vi "myRIO Main v2.vi"() -> ()   [LabVIEW 2014]
uses:
  Type Defs/VL6180 states.ctl
  <vilib>/Platform/TimedLoop/XDataNode/timing_clust.ctl
  <vilib>/Platform/TimedLoop/XDataNode/nitl_modes.ctl
  <vilib>/Platform/TimedLoop/XDataNode/wakeup.ctl
  Type Defs/VL6180 Resource.ctl
  <vilib>/myRIO/Instrument Drivers/Onboard IO/DIO/typedefs/DIO Reference.ctl
  <vilib>/myRIO/Common/Instrument Driver Framework/Utilities/typedefs/myRIO Generic Hardware Reference.ctl
  <vilib>/myRIO/Common/Instrument Driver Framework/Utilities/typedefs/Hardware Version Enum.ctl
  <vilib>/myRIO/Common/Instrument Driver Framework/Utilities/typedefs/myRIO v1.0 Reference.ctl
  <vilib>/myRIO/Common/Instrument Driver Framework/Utilities/typedefs/Generic FPGA Reference.ctl
  <vilib>/myRIO/Common/Instrument Driver Framework/myRIO v1.0/DIO/typedefs/DIO Channels List.ctl
  <vilib>/myRIO/Common/Instrument Driver Framework/myRIO v1.0/DIO/typedefs/DIO Channels Enum.ctl
  <vilib>/userdefined/High Color/nirio_resource_hc.ctl
  <vilib>/myRIO/Instrument Drivers/Onboard IO/AI/typedefs/AI Reference.ctl
  <vilib>/myRIO/Common/Instrument Driver Framework/myRIO v1.0/AI/typedefs/AI Channels List.ctl
  <vilib>/myRIO/Common/Instrument Driver Framework/myRIO v1.0/AI/typedefs/AI Channels Enum.ctl
  <vilib>/myRIO/Common/Instrument Driver Framework/Utilities/typedefs/Analog Scaling Constants List.ctl
  <vilib>/myRIO/Common/Instrument Driver Framework/Utilities/typedefs/Analog Scaling Constants.ctl
  <vilib>/myRIO/Common/Instrument Driver Framework/Utilities/vis/Is FPGA Ref Available.vi
  <vilib>/myRIO/Common/Instrument Driver Framework/myRIO v1.0/DIO/vis/myRIO v1.1 Open DIO.vi
  <vilib>/myRIO/Instrument Drivers/Onboard IO/DIO/vis/Read.vi
  <vilib>/myRIO/Common/Instrument Driver Framework/myRIO v1.0/AI/vis/myRIO v1.1 Open AI.vi
  <vilib>/myRIO/Instrument Drivers/Onboard IO/AI/vis/Read.vi
  <vilib>/myRIO/Instrument Drivers/Onboard IO/DIO/vis/Write.vi
  <vilib>/MakerHub/LINX/Public/Peripherals/Digital/Digital Write 1 Chan.vi
  <vilib>/myRIO/Common/Instrument Driver Framework/Utilities/vis/Validate Channels.vi
  <vilib>/myRIO/Common/Instrument Driver Framework/myRIO v1.0/DIO/vis/myRIO v1.0 Reserve DIO.vi
  <vilib>/myRIO/Common/Instrument Driver Framework/myRIO v1.0/AI/vis/myRIO v1.0 Reserve AI.vi
  <vilib>/MakerHub/LINX/Public/Peripherals/Digital/Digital Write N Chans.vi
  <vilib>/myRIO/Common/Instrument Driver Framework/myRIO v1.0/Resource Manager/vis/myRIO v1.0 Reserve Channel List.vi
  <vilib>/myRIO/Common/Instrument Driver Framework/myRIO v1.0/DIO/vis/myRIO v1.0 Build MUX Configuration DIO.vi
  <vilib>/myRIO/Common/Instrument Driver Framework/myRIO v1.0/AI/vis/myRIO v1.0 Build MUX Configuration AI.vi
  <vilib>/MakerHub/LINX/Private/Local IO/LinxDigitalWrite.vi
  <vilib>/MakerHub/LINX/Public/Utilities/Check Channel.vi
  <vilib>/myRIO/Common/Instrument Driver Framework/myRIO v1.0/Resource Manager/vis/myRIO v1.0 Reserve Channel.vi
  <vilib>/myRIO/Common/Instrument Driver Framework/myRIO v1.0/Resource Manager/vis/myRIO v1.0 Unreserve Channel.vi
  <vilib>/myRIO/Common/Instrument Driver Framework/myRIO v1.0/Resource Manager/vis/myRIO v1.0 Create Configuration List.vi
  <vilib>/MakerHub/LINX/Private/myRIO/Utilities/Get DIO Channel Name.vi
  <vilib>/myRIO/Common/Instrument Driver Framework/myRIO v1.0/Resource Manager/vis/myRIO v1.0 Build Mutex Name.vi
  <vilib>/Utility/VariantDataType/GetNumericInfo.vi
  <vilib>/Utility/error.llb/Error Cluster From Error Code.vi
  <vilib>/myRIO/Common/Instrument Driver Framework/myRIO v1.0/myRIO v1.1 Open.vi
  <vilib>/myRIO/Common/Instrument Driver Framework/myRIO v1.0/AI/vis/myRIO v1.0 Get Scaling Constants AI.vi
  <vilib>/myRIO/Common/Instrument Driver Framework/Utilities/vis/IO Manager.vi
  <vilib>/myRIO/Common/Instrument Driver Framework/Utilities/vis/Configuration Manager.vi
  <vilib>/myRIO/Common/Instrument Driver Framework/myRIO v1.0/myRIO v1.0 Close.vi
  <vilib>/myRIO/Common/Instrument Driver Framework/myRIO v1.0/AI/vis/myRIO v1.0 Read AI.vi
  <vilib>/myRIO/Common/Instrument Driver Framework/myRIO v1.0/Resource Manager/vis/myRIO v1.0 Configure IO.vi
  <vilib>/myRIO/Common/Instrument Driver Framework/myRIO v1.0/DIO/vis/myRIO v1.0 Write DIO.vi
  <vilib>/MakerHub/LINX/Public/Utilities/Open Local.vi
  <vilib>/MakerHub/LINX/Private/Utilties/Generate Error.vi
  <vilib>/myRIO/Instrument Drivers/Onboard IO/DIO/vis/Smart Open.vi
  <vilib>/myRIO/Common/Instrument Driver Framework/myRIO v1.0/DIO/vis/myRIO v1.0 Read DIO.vi
  <vilib>/myRIO/Express VI/Onboard IO/AI/AI Express VI.xnode
  <vilib>/myRIO/Instrument Drivers/Onboard IO/AI/vis/myRIO AI Open.xnode
  <vilib>/myRIO/Express VI/Onboard IO/DO/DO Express VI.xnode
  <vilib>/myRIO/Instrument Drivers/Onboard IO/DIO/vis/myRIO DIO Open.xnode
  <vilib>/platform/TimedLoop/XDataNode/XDataNode.xnode
  <vilib>/myRIO/Express VI/Onboard IO/DI/DI Express VI.xnode
  <vilib>/MakerHub/LINX/LMH-LINX.lvlib
  <vilib>/Platform/TimedLoop/XDataNode/XDNodeRunTimeDep.lvlib
  <vilib>/myRIO/Instrument Drivers/Onboard IO/DIO/DIO.lvlib
  <vilib>/myRIO/Express VI/Onboard IO/I2C/I2C Express VI.xnode
  <vilib>/myRIO/Instrument Drivers/Onboard IO/I2C/vis/Configure.vi
  <vilib>/myRIO/Instrument Drivers/Onboard IO/I2C/I2C.lvlib
  <vilib>/myRIO/Instrument Drivers/Onboard IO/I2C/vis/Write.vi
  <vilib>/myRIO/Instrument Drivers/Onboard IO/I2C/typedefs/I2C Transfer Rate.ctl
  <vilib>/myRIO/Instrument Drivers/Onboard IO/I2C/typedefs/I2C User Configuration.ctl
  <vilib>/myRIO/Instrument Drivers/Onboard IO/I2C/typedefs/I2C Configuration.ctl
  <vilib>/myRIO/Common/Instrument Driver Framework/myRIO v1.0/I2C/typedefs/I2C Channels Enum.ctl
  <vilib>/myRIO/Instrument Drivers/Onboard IO/I2C/typedefs/I2C Reference.ctl
  <vilib>/myRIO/Instrument Drivers/Onboard IO/I2C/vis/myRIO I2C Open.xnode
  <vilib>/myRIO/Common/Instrument Driver Framework/myRIO v1.0/I2C/vis/myRIO v1.1 Open I2C.vi
  <vilib>/myRIO/Instrument Drivers/Onboard IO/I2C/vis/Read.vi
  <vilib>/myRIO/Instrument Drivers/Onboard IO/AI/AI.lvlib
panel:
  out "5V Regulator":dbl(knob) scale=0.0..6.0
  in  "Sensor Power":bool
  out "Laser Error":bool
  in  "Reset":bool
  in  "Stop":bool
  in  "Wait (ms)":u32=10
  out "ToF Loop Rate":u32
  in  "Speed Read":bool
  out "Attempts":i32
  out "Sensor Error Code":u8
  in  "Attempts before Timeout":u16=10
  in  "delay":u32=500
  in  "I2C Channel":u8
  out "Sensors Online":bool[](array[boolean])
  in  "# of sensors":i32=5
  out "Status":string
  in  "Track Location":dbl(slide) scale=0.0..5000.0
  out "Structure\nStress":dbl(slide) scale=2.4..2.6
  out "Track Position":T1
  out "Battery (Primary)":dbl(slide) scale=0.0..100.0 scale format="%.1f%"
  out "Current":dbl(knob) scale=0.0..1.0
  out "IMU":T2 {"Magnetometer"."Z" scale=0.0..100.0; "Magnetometer"."Y" scale=0.0..100.0; "Magnetometer"."X" scale=0.0..100.0; "Gyroscope"."R" scale=0.0..100.0; "Gyroscope"."Y" scale=0.0..100.0; "Gyroscope"."P" scale=0.0..100.0; "Accelerometer"."Z" scale=0.0..100.0; "Accelerometer"."Y" scale=0.0..100.0; "Accelerometer"."X" scale=0.0..100.0}
  out "Voltage":dbl(knob) scale=0.0..12.0
  out "Gap 4":u8(slide) scale=0.0..100.0
  out "Gap 3":u8(slide) scale=0.0..100.0
  out "Rail Gap 2":u8(slide) scale=0.0..100.0
  out "Gap 2":u8(slide) scale=0.0..100.0
  out "Temp 2":dbl(slide) scale=0.0..100.0
  out "Temp 1":dbl(slide) scale=0.0..100.0
  out "Rail Gap 1":u8(slide) scale=0.0..100.0
  out "Gap 1":u8(slide) scale=0.0..100.0
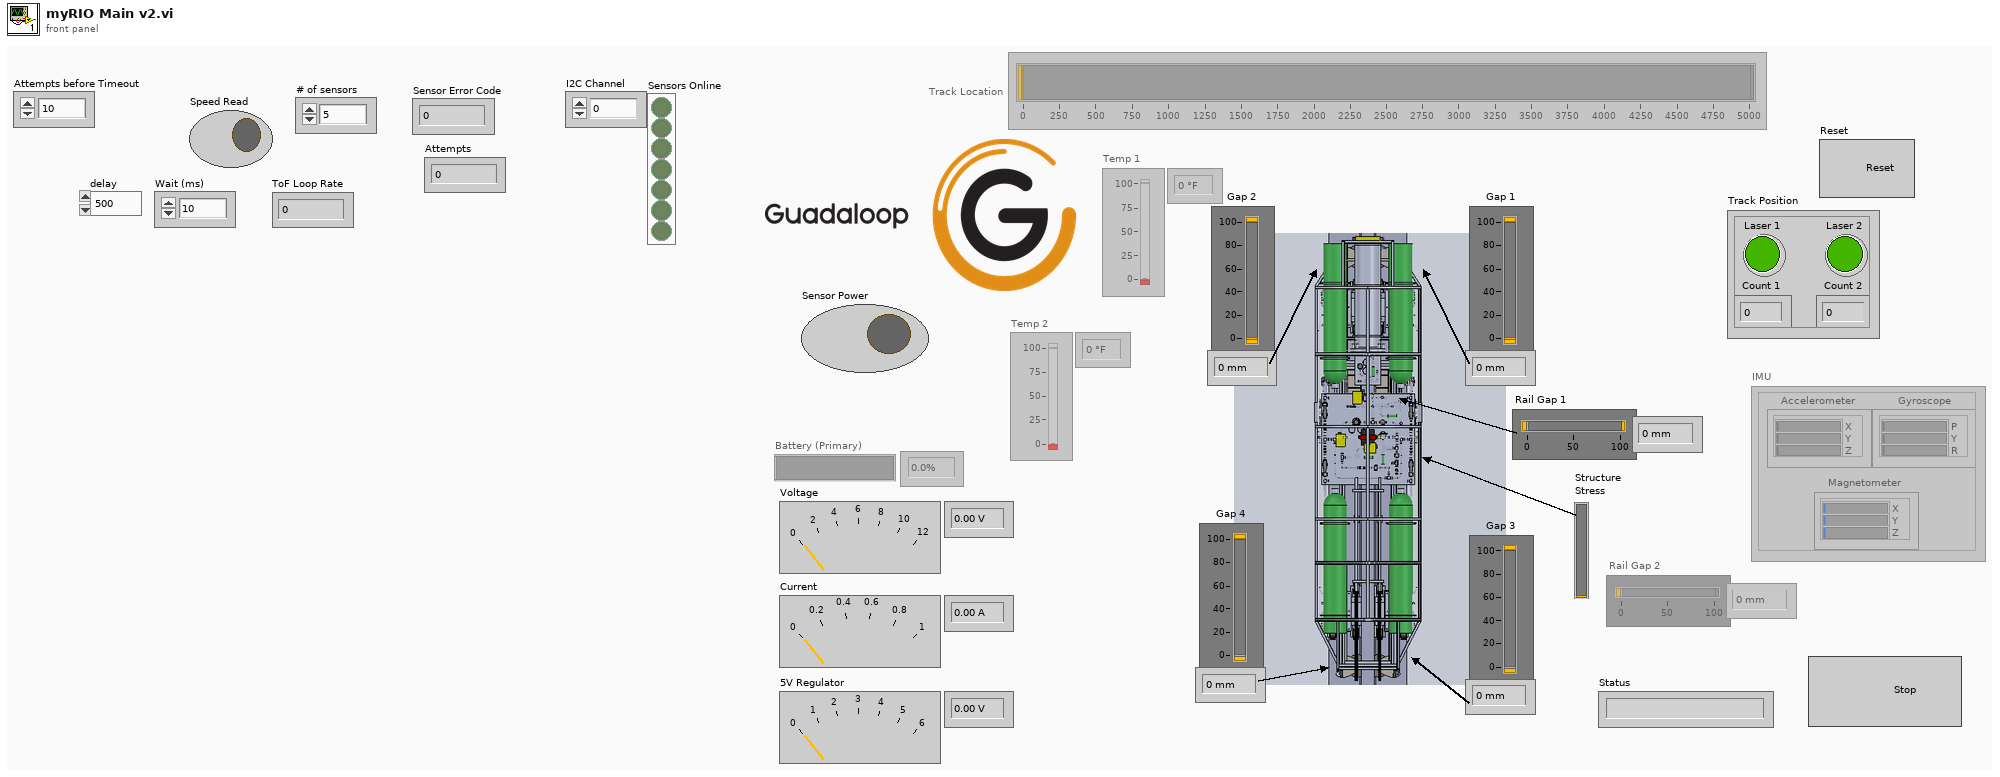
[diagram p1: front panel]
types:
  T1 = cluster{"Laser 1":bool, "Count 1":u32, "Laser 2":bool, "Count 2":u32}
  T2 = cluster{"Accelerometer":cluster{"X":u8, "Y":u8, "Z":u8}, "Gyroscope":cluster{"P":u8, "Y":u8, "R":u8}, "Magnetometer":cluster{"X":u8, "Y":u8, "Z":u8}}
  T3 = typedef "VL6180 states.ctl" = enum16{"Ping All", "Initialize", "Read"}
  T4 = typedef "XDNodeRunTimeDep.lvlib/timing_clust.ctl" = cluster{"Expected End [f-1]":u64, "Actual End [f-1]":u64, "Finished Late? [f-1]":bool, "Expected End [i-1]":u64, "Actual End [i-1]":u64, "Finished Late? [i-1]":bool, "Expected Start [i]":u64, "Actual Start [i]":u64, "Expected Start [f]":u64, "Actual Start [f]":u64, "Source Name":string, "Structure Name":string, "Period":i64, "Deadline":i64, "Offset":i64, "Start":i64, "Priority":i32, "Timeout":i32, "Mode":T5, "Wakeup Reason":T6, "Error":errorcluster, "Source Type":string, "Secondary Source Type":string, "Global End Time":u64, "Global Start Time":u64, "Frame Duration":u64, "Iteration Duration":u64, "Assigned CPU":i32, "I/O Scan Engine Mode":u32}
  T5 = typedef "XDNodeRunTimeDep.lvlib/nitl_modes.ctl" = enum32{"No Change", "Process missed periods, maintain original phase", "Discard missed periods, maintain original phase", "Process missed periods, ignore original phase", "Discard missed periods, ignore original phase"}
  T6 = typedef "XDNodeRunTimeDep.lvlib/wakeup.ctl" = enum32{"Normal", "Aborted", "Asynchronous wakeup", "Timing source error", "Timed loop error", "Timeout"}
  T7 = typedef "LMH-LINX.lvlib/LINX Ref.ctl" = cluster{"IO":T8, "Interface":T9, "LINX Device Config":T10}
  T8 = typedef "LMH-LINX.lvlib/Platform.ctl" = enum16{"Remote", "Local"}
  T9 = typedef "LMH-LINX.lvlib/Interface.ctl" = enum16{"Serial", "TCP"}
  T10 = typedef "LMH-LINX.lvlib/Device.lvlib/LINX Device Config.ctl" = cluster{"Interface":T9, "COM Port":refnum<visa-resource-name>, "TCP Configuration":T11, "Device Family":u8, "Device ID":u8, "Device Name":string, "TCP Ref":refnum<k5>, "Channels":T12}
  T11 = typedef "LMH-LINX.lvlib/Device.lvlib/TCP Config.ctl" = cluster{"IP Address":string, "Port":u16}
  T12 = typedef "LMH-LINX.lvlib/Channels.ctl" = cluster{"DI":u8[], "DO":u8[], "AI":u8[], "AO":u8[], "PWM":u8[], "QE":u8[], "UART":u8[], "I2C 2":u8[], "SPI":u8[], "CAN":u8[], "Servo":u8[], "AI Ref (V)":dbl, "AI Resolution (Bits)":u8, "AO Ref (V)":dbl, "AO Resolution (Bits)":u8}
  T13 = typedef "DIO.lvlib/DIO Reference.ctl" = cluster{"myRIO Reference":T14, "DIO Channels List":T18}
  T14 = typedef "myRIO Generic Hardware Reference.ctl" = cluster{"myRIO Model":T15, "myRIO Hardware Reference":T16}
  T15 = typedef "Hardware Version Enum.ctl" = enum16{"Unknown", "myRIO-1900", "myRIO-1950"}
  T16 = typedef "myRIO v1.0 Reference.ctl" = cluster{"Generic FPGA Reference":T17, "Allow multiple opens":bool}
  T17 = typedef "Generic FPGA Reference.ctl" = refnum<k20>
  T18 = typedef "DIO Channels List.ctl" = T19[]
  T19 = typedef "DIO Channels Enum.ctl" = enum16{"Not Connected", "C/DIO0", "C/DIO1", "C/DIO2", "C/DIO3", "C/DIO4", "C/DIO5", "C/DIO6", "C/DIO7", "A/DIO0", "A/DIO1", "A/DIO2", "A/DIO3", "A/DIO4", "A/DIO5", "A/DIO6", "A/DIO7", "A/DIO8", "A/DIO9", "A/DIO10", "A/DIO11", "A/DIO12", "A/DIO13", "A/DIO14", "A/DIO15", "B/DIO0", "B/DIO1", "B/DIO2", "B/DIO3", "B/DIO4", "B/DIO5", "B/DIO6", "B/DIO7", "B/DIO8", "B/DIO9", "B/DIO10", "B/DIO11", "B/DIO12", "B/DIO13", "B/DIO14", "B/DIO15", "LED0", "LED1", "LED2", "LED3", "Button0"}
  T20 = typedef "nirio_resource_hc.ctl" = tag
  T21 = typedef "VL6180 Resource.ctl" = cluster{"I2C Channel":u8, "I2C Slave Address":u8, "Online":bool}
  T22 = typedef "I2C.lvlib/I2C Reference.ctl" = cluster{"myRIO Reference":T14, "I2C Channels Enum":T23, "I2C Configuration":T24}
  T23 = typedef "I2C Channels Enum.ctl" = enum16{"Not Connected", "A/I2C", "B/I2C"}
  T24 = typedef "I2C.lvlib/I2C Configuration.ctl" = cluster{"I2C Transfer Rate":T25}
  T25 = typedef "I2C.lvlib/I2C Transfer Rate.ctl" = enum16{"Standard mode (100 kbps)", "Fast mode (400 kbps)"}
  T26 = typedef "I2C.lvlib/I2C User Configuration.ctl" = cluster{"I2C Transfer Rate":T25}
  T27 = typedef "AI.lvlib/AI Reference.ctl" = cluster{"myRIO Reference":T14, "AI Channels List":T28, "AI Scaling Constants List":T30}
  T28 = typedef "AI Channels List.ctl" = T29[]
  T29 = typedef "AI Channels Enum.ctl" = enum16{"Not Connected", "AudioIn/Left", "AudioIn/Right", "C/AI0", "C/AI1", "A/AI0", "A/AI1", "A/AI2", "A/AI3", "B/AI0", "B/AI1", "B/AI2", "B/AI3"}
  T30 = typedef "Analog Scaling Constants List.ctl" = T31[]
  T31 = typedef "Analog Scaling Constants.ctl" = cluster{"LSB Weight (Volts)":dbl, "Offset (Volts)":dbl, "Signed?":bool}
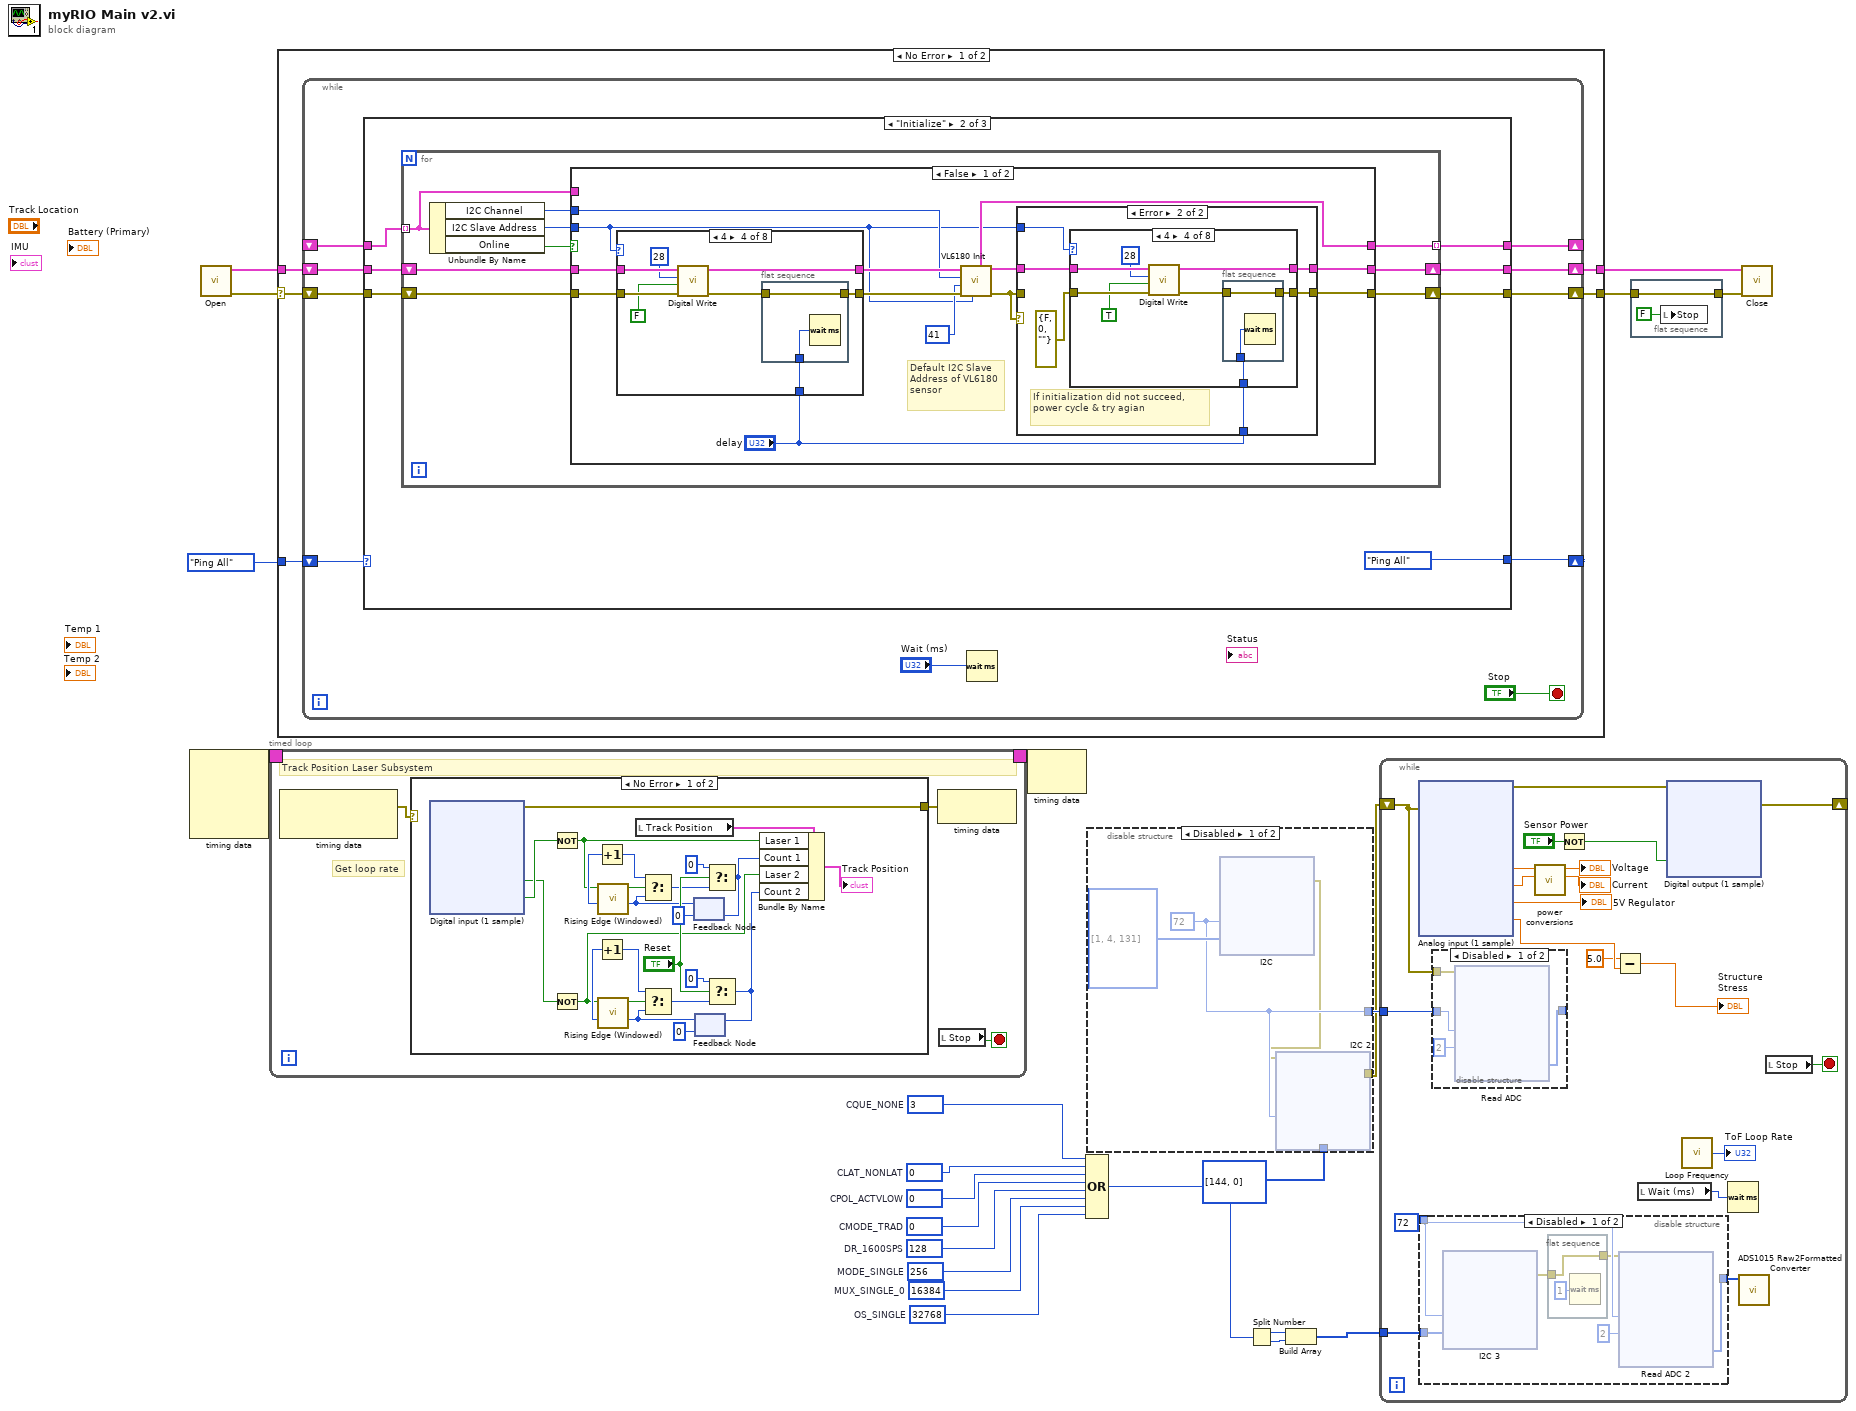
[diagram p0: block diagram]
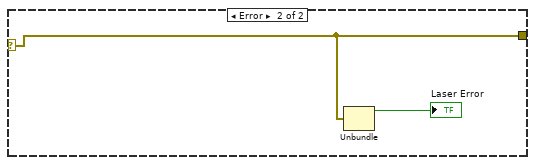
[diagram p5: hidden frame]
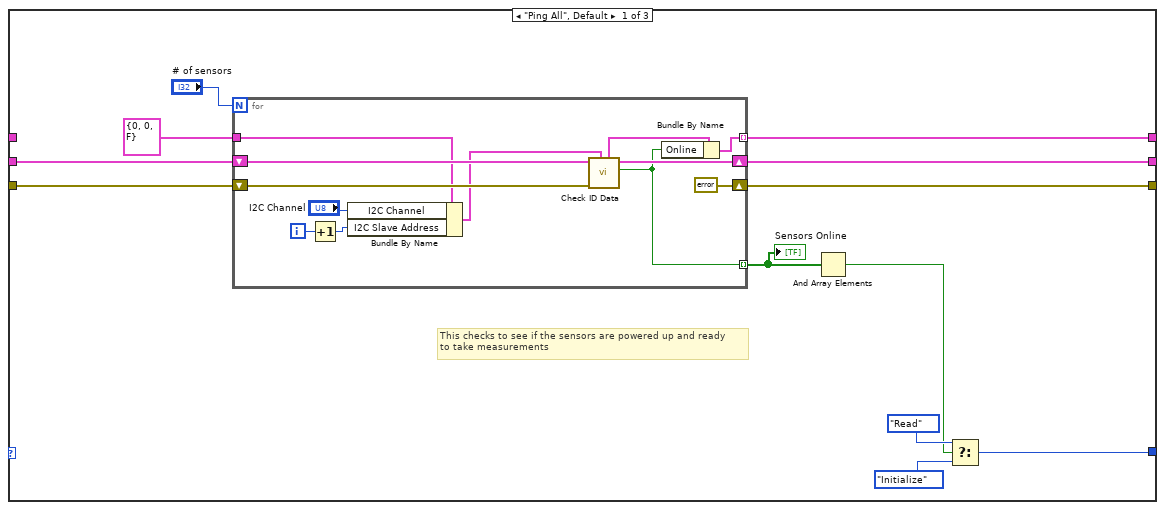
[diagram p6: hidden frame]
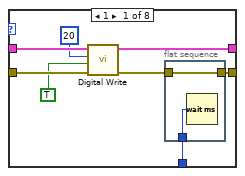
[diagram p8: hidden frame]
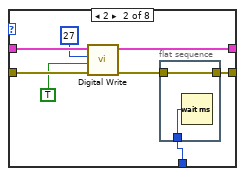
[diagram p9: hidden frame]
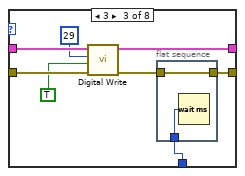
[diagram p10: hidden frame]
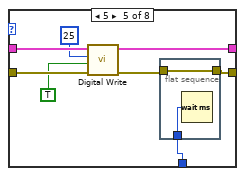
[diagram p11: hidden frame]
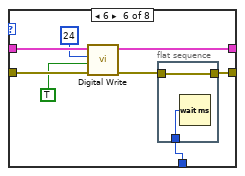
[diagram p12: hidden frame]
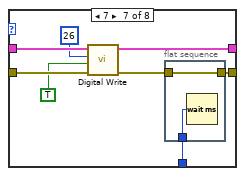
[diagram p13: hidden frame]
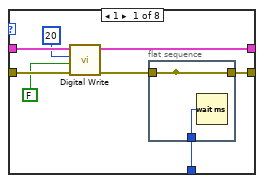
[diagram p15: hidden frame]
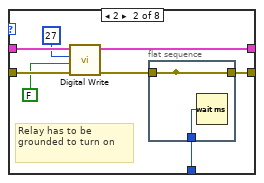
[diagram p16: hidden frame]
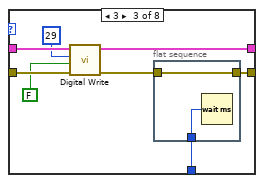
[diagram p17: hidden frame]
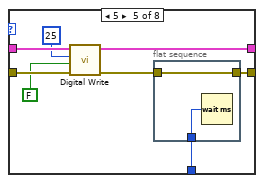
[diagram p18: hidden frame]
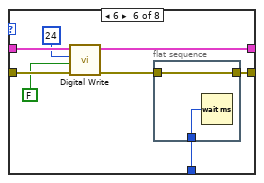
[diagram p19: hidden frame]
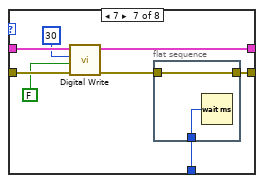
[diagram p20: hidden frame]
diagram:
  w5 = u16 32768  # OS_SINGLE
  w6 = u16 16384  # MUX_SINGLE_0
  w7 = u16 256  # MODE_SINGLE
  w8 = u16 128  # DR_1600SPS
  w9 = u16 0  # CMODE_TRAD
  w10 = u16 0  # CPOL_ACTVLOW
  w11 = u16 0  # CLAT_NONLAT
  w12 = u16 3  # CQUE_NONE
  n1 = node-c288() -> (w19:T4)  [unwired: 4 in]
  n2 = call-poly <vilib>:"Open.vi"() -> ("Error Out"=w22:errorcluster, "LINX Resource"=w23:T7)  [unwired: 9 in, 1 out]
  n3 = timed-loop {
    timing: w19 -> [_]
    timing-out: [_] -> w18
    stop <- w26 stop-if-true
    # "Get loop rate"
    # "Track Position Laser Subsystem"
    n4 = node-c288() -> (w25:errorcluster)  [unwired: 1 in, 1 out]
    n5 = case shown="No Error" w25 {
      selector: w25 -> [_ w86]
      tunnel: [w31 w86] -> w24
      frame No Error {
        n6 = xnode "Digital input (1 sample)"() -> ("Laser 1 (A/DIO0 (Pin 11))"=w27:bool, "Laser 2 (A/DIO1 (Pin 13))"=w28:bool, "error out"=w31:errorcluster)  [unwired: 1 in]
        n7 = Not(x=w28) -> (.not. x?=w36:bool)
        n8 = Not(x=w27) -> (.not. x?=w33:bool)
        n9 = call "Rising Edge (Windowed).vi"("Input"=w36) -> ("Rising Edge?"=w41:bool)  [unwired: 10 in]
        n10 = call "Rising Edge (Windowed).vi"("Input"=w33) -> ("Rising Edge?"=w34:bool)  [unwired: 10 in]
        n11 = local read "Track Position"() -> (w38:T1)
        n12 = feedback #1(u32 0 ("t")) -> (w40:u32)
        n13 = Increment(x=w40) -> (x+1=w42:u32)
        n14 = Select(t=w42, s=w41, f=w40) -> (s? t:f=w43:u32)
        n15 = feedback #2(u32 0 ("t")) -> (w39:u32)
        n16 = Increment(x=w39) -> (x+1=w45:u32)
        n17 = Select(t=w45, s=w34, f=w39) -> (s? t:f=w46:u32)
        n18 = Select(t=u32 0, s="Reset", f=w43) -> (s? t:f=w35:u32)
        n19 = feedback-in #1(w35) -> ()
        n20 = Select(t=u32 0, s="Reset", f=w46) -> (s? t:f=w32:u32)
        n21 = feedback-in #2(w32) -> ()
        n22 = Bundle By Name(cluster=w38, "Laser 1"=w36, "Count 1"=w35, "Laser 2"=w33, "Count 2"=w32) -> (→"Track Position":T1)
      }
      frame Error {
        n23 = Unbundle(w86) -> ("status"=→"Laser Error":bool)  [unwired: 2 out]
      }
    }
    n24 = node-c288(w24) -> ()  [unwired: 1 out]
    n25 = local read "Stop"() -> (w26:bool)
  }
  n26 = case shown="No Error" w22 {
    selector: w22 -> [w94 w349]
    tunnel: [w96 w349] -> w17
    tunnel: [w95 w348] -> w20
    tunnel: VL6180_states."Ping All" -> [w93 _]
    tunnel: w23 -> [w92 w348]
    frame No Error {
      n27 = while {
        shift-right: [w98] -> w95
        shift-left: w92 -> [w104]
        shift-right: [w97] -> w96
        shift-left: w94 -> [w103]
        shift-right: [w99] -> _
        shift-left: _ -> [w102]
        shift-right: [w100] -> _
        shift-left: w93 -> [w101]
        stop <- "Stop" stop-if-true
        n28 = case shown="\"Initialize\"" w101 {
          tunnel: w104 -> [w118 w137 w334]
          tunnel: w103 -> [w117 w131 w336]
          tunnel: w102 -> [_ w135 w333]
          tunnel: [w115 w132 w335] -> w99
          tunnel: [w116 w134 w328] -> w98
          tunnel: [w110 VL6180_states."Ping All" w332] -> w100
          tunnel: [w109 w133 w327] -> w97
          frame "Ping All", Default {
            # "This checks to see if the sensors are powered up and ready\nto take measurements"
            n29 = for {
              N: "# of sensors" -> [_]
              tunnel: T21 {"I2C Channel"=0, "I2C Slave Address"=0, "Online"=FALSE} ("VL6180 Resource out") -> [w123]
              shift-right: [w126] -> w116
              shift-left: w118 -> [w130]
              tunnel: [w125] -> w115 mode=indexing
              tunnel: [w124] -> w114 mode=indexing
              shift-right: [errorcluster {"status"=FALSE, "code"=0, "source"=""} ("error IO")] -> w109
              shift-left: w117 -> [w129]
              i -> [w127]
              n30 = Increment(x=w127) -> (x+1=w120:i32)
              n31 = Bundle By Name(cluster=w123, "I2C Channel"="I2C Channel", "I2C Slave Address"=w120) -> (w122:T21)
              n32 = call "Check ID Data.vi"("VL6180 Resource"=w122, "Error In"=w129, "LINX Resource"=w130) -> ("Same Model?"=w124:bool, "LINX Resource"=w126:T7, "VL6180 Resource"=w128:T21)  [unwired: 5 in, 1 out]
              n33 = Bundle By Name(cluster=w128, "Online"=w124) -> (w125:T21)
            }
            "Sensors Online" <- w114
            n34 = And Array Elements(Boolean array=w114) -> (logical AND=w111:bool)
            n35 = Select(t=VL6180_states."Read", s=w111, f=VL6180_states."Initialize") -> (s? t:f=w110:T3)
          }
          frame "Initialize" {
            n36 = for {
              tunnel: w135 -> [w138] mode=indexing
              shift-right: [w145] -> w134
              shift-left: w137 -> [w146]
              shift-right: [w144] -> w133
              shift-left: w131 -> [w140]
              tunnel: [w141] -> w132 mode=indexing
              n37 = Unbundle By Name(w138) -> ("I2C Channel"=w143:u8, "I2C Slave Address"=w142:u8, "Online"=w139:bool)
              n38 = case shown="False" w139 {
                tunnel: w146 -> [w159 w315]
                tunnel: w140 -> [w156 w314]
                tunnel: [w153 w315] -> w145
                tunnel: [w152 w314] -> w144
                tunnel: w143 -> [w148 _]
                tunnel: w142 -> [w147 _]
                tunnel: [w154 w313] -> w141
                tunnel: w138 -> [_ w313]
                frame False {
                  # "Default I2C Slave Address of VL6180 sensor"
                  n39 = case shown="4" w147 {
                    tunnel: w159 -> [w247 w257 w267 w277 w287 w297 w307 w311]
                    tunnel: [w246 w256 w266 w276 w286 w296 w306 w311] -> w158
                    tunnel: [w242 w252 w261 w271 w281 w291 w301 w310] -> w157
                    tunnel: w156 -> [w245 w255 w265 w275 w285 w295 w305 w310]
                    tunnel: "delay" -> [w240 w250 w260 w270 w280 w290 w300 _]
                    frame 1 {
                      n40 = call-poly <vilib>:"Digital Write.vi"("Error In"=w245, "Output Value"=FALSE, "DO Channel"=u8 20, "LINX Resource"=w247) -> ("Error Out"=w241:errorcluster, "LINX Resource"=w246:T7)  [unwired: 6 in]
                      n41 = flat-sequence {
                        tunnel: [w249] -> _
                        tunnel: [w249] -> w242
                        tunnel: w241 -> [w249]
                        tunnel: w240 -> [w248]
                        frame #0 {
                          n42 = Wait (ms)(milliseconds to wait=w248) -> ()  [unwired: 1 out]
                        }
                      }
                    }
                    frame 2 {
                      # "Relay has to be grounded to turn on"
                      n43 = call-poly <vilib>:"Digital Write.vi"("Error In"=w255, "Output Value"=FALSE, "DO Channel"=u8 27, "LINX Resource"=w257) -> ("Error Out"=w251:errorcluster, "LINX Resource"=w256:T7)  [unwired: 6 in]
                      n44 = flat-sequence {
                        tunnel: [w259] -> _
                        tunnel: [w259] -> w252
                        tunnel: w251 -> [w259]
                        tunnel: w250 -> [w258]
                        frame #0 {
                          n45 = Wait (ms)(milliseconds to wait=w258) -> ()  [unwired: 1 out]
                        }
                      }
                    }
                    frame 3 {
                      n46 = call-poly <vilib>:"Digital Write.vi"("Error In"=w265, "Output Value"=FALSE, "DO Channel"=u8 29, "LINX Resource"=w267) -> ("Error Out"=w262:errorcluster, "LINX Resource"=w266:T7)  [unwired: 6 in]
                      n47 = flat-sequence {
                        tunnel: w262 -> [w269]
                        tunnel: [w269] -> w261
                        tunnel: w260 -> [w268]
                        frame #0 {
                          n48 = Wait (ms)(milliseconds to wait=w268) -> ()  [unwired: 1 out]
                        }
                      }
                    }
                    frame 4 {
                      n49 = call-poly <vilib>:"Digital Write.vi"("Error In"=w275, "Output Value"=FALSE, "DO Channel"=u8 28, "LINX Resource"=w277) -> ("Error Out"=w272:errorcluster, "LINX Resource"=w276:T7)  [unwired: 6 in]
                      n50 = flat-sequence {
                        tunnel: w272 -> [w279]
                        tunnel: [w279] -> w271
                        tunnel: w270 -> [w278]
                        frame #0 {
                          n51 = Wait (ms)(milliseconds to wait=w278) -> ()  [unwired: 1 out]
                        }
                      }
                    }
                    frame 5 {
                      n52 = call-poly <vilib>:"Digital Write.vi"("Error In"=w285, "Output Value"=FALSE, "DO Channel"=u8 25, "LINX Resource"=w287) -> ("Error Out"=w282:errorcluster, "LINX Resource"=w286:T7)  [unwired: 6 in]
                      n53 = flat-sequence {
                        tunnel: w282 -> [w289]
                        tunnel: [w289] -> w281
                        tunnel: w280 -> [w288]
                        frame #0 {
                          n54 = Wait (ms)(milliseconds to wait=w288) -> ()  [unwired: 1 out]
                        }
                      }
                    }
                    frame 6 {
                      n55 = call-poly <vilib>:"Digital Write.vi"("Error In"=w295, "Output Value"=FALSE, "DO Channel"=u8 24, "LINX Resource"=w297) -> ("Error Out"=w292:errorcluster, "LINX Resource"=w296:T7)  [unwired: 6 in]
                      n56 = flat-sequence {
                        tunnel: w292 -> [w299]
                        tunnel: [w299] -> w291
                        tunnel: w290 -> [w298]
                        frame #0 {
                          n57 = Wait (ms)(milliseconds to wait=w298) -> ()  [unwired: 1 out]
                        }
                      }
                    }
                    frame 7 {
                      n58 = call-poly <vilib>:"Digital Write.vi"("Error In"=w305, "Output Value"=FALSE, "DO Channel"=u8 30, "LINX Resource"=w307) -> ("Error Out"=w302:errorcluster, "LINX Resource"=w306:T7)  [unwired: 6 in]
                      n59 = flat-sequence {
                        tunnel: w302 -> [w309]
                        tunnel: [w309] -> w301
                        tunnel: w300 -> [w308]
                        frame #0 {
                          n60 = Wait (ms)(milliseconds to wait=w308) -> ()  [unwired: 1 out]
                        }
                      }
                    }
                    frame 9, Default {
                      n61 = local write "Status"("Plug new sensor in" ("message")) -> ()
                    }
                  }
                  n62 = call "VL6180 Init.vi"("Change Slave Address"=w147, "Error In"=w157, "I2C Slave Address (0)"=u8 41, "I2C Channel"=w148, "LINX Resource"=w158) -> ("Error Out"=w150:errorcluster, "LINX Resource"=w151:T7, "VL6180 Resource"=w154:T21)  [unwired: 4 in]
                  n63 = case shown="Error" w150 {
                    tunnel: [w161 w167] -> w153
                    tunnel: [w160 w164] -> w152
                    tunnel: w151 -> [w161 w166]
                    tunnel: w150 -> [w160 _]
                    tunnel: "delay" -> [_ w163]
                    tunnel: w147 -> [_ w162]
                    frame No Error {
                      # "Initialization successful"
                    }
                    frame Error {
                      # "If initialization did not succeed, power cycle & try agian"
                      n64 = case shown="4" w162 {
                        tunnel: w166 -> [w175 w185 w195 w205 w215 w225 w235 w239]
                        tunnel: [w174 w184 w194 w204 w214 w224 w234 w239] -> w167
                        tunnel: [w169 w178 w189 w199 w209 w219 w229 w238] -> w164
                        tunnel: errorcluster {"status"=FALSE, "code"=0, "source"=""} ("Error Out") -> [w173 w183 w193 w203 w213 w223 w233 w238]
                        tunnel: w163 -> [w168 w179 w188 w198 w208 w218 w228 _]
                        frame 1 {
                          n65 = call-poly <vilib>:"Digital Write.vi"("Error In"=w173, "Output Value"=TRUE, "DO Channel"=u8 20, "LINX Resource"=w175) -> ("Error Out"=w170:errorcluster, "LINX Resource"=w174:T7)  [unwired: 6 in]
                          n66 = flat-sequence {
                            tunnel: [w177] -> w169
                            tunnel: w170 -> [w177]
                            tunnel: w168 -> [w176]
                            frame #0 {
                              n67 = Wait (ms)(milliseconds to wait=w176) -> ()  [unwired: 1 out]
                            }
                          }
                        }
                        frame 2 {
                          n68 = call-poly <vilib>:"Digital Write.vi"("Error In"=w183, "Output Value"=TRUE, "DO Channel"=u8 27, "LINX Resource"=w185) -> ("Error Out"=w180:errorcluster, "LINX Resource"=w184:T7)  [unwired: 6 in]
                          n69 = flat-sequence {
                            tunnel: [w187] -> w178
                            tunnel: w180 -> [w187]
                            tunnel: w179 -> [w186]
                            frame #0 {
                              n70 = Wait (ms)(milliseconds to wait=w186) -> ()  [unwired: 1 out]
                            }
                          }
                        }
                        frame 3 {
                          n71 = call-poly <vilib>:"Digital Write.vi"("Error In"=w193, "Output Value"=TRUE, "DO Channel"=u8 29, "LINX Resource"=w195) -> ("Error Out"=w190:errorcluster, "LINX Resource"=w194:T7)  [unwired: 6 in]
                          n72 = flat-sequence {
                            tunnel: [w197] -> w189
                            tunnel: w190 -> [w197]
                            tunnel: w188 -> [w196]
                            frame #0 {
                              n73 = Wait (ms)(milliseconds to wait=w196) -> ()  [unwired: 1 out]
                            }
                          }
                        }
                        frame 4 {
                          n74 = call-poly <vilib>:"Digital Write.vi"("Error In"=w203, "Output Value"=TRUE, "DO Channel"=u8 28, "LINX Resource"=w205) -> ("Error Out"=w200:errorcluster, "LINX Resource"=w204:T7)  [unwired: 6 in]
                          n75 = flat-sequence {
                            tunnel: [w207] -> w199
                            tunnel: w200 -> [w207]
                            tunnel: w198 -> [w206]
                            frame #0 {
                              n76 = Wait (ms)(milliseconds to wait=w206) -> ()  [unwired: 1 out]
                            }
                          }
                        }
                        frame 5 {
                          n77 = call-poly <vilib>:"Digital Write.vi"("Error In"=w213, "Output Value"=TRUE, "DO Channel"=u8 25, "LINX Resource"=w215) -> ("Error Out"=w210:errorcluster, "LINX Resource"=w214:T7)  [unwired: 6 in]
                          n78 = flat-sequence {
                            tunnel: [w217] -> w209
                            tunnel: w210 -> [w217]
                            tunnel: w208 -> [w216]
                            frame #0 {
                              n79 = Wait (ms)(milliseconds to wait=w216) -> ()  [unwired: 1 out]
                            }
                          }
                        }
                        frame 6 {
                          n80 = call-poly <vilib>:"Digital Write.vi"("Error In"=w223, "Output Value"=TRUE, "DO Channel"=u8 24, "LINX Resource"=w225) -> ("Error Out"=w220:errorcluster, "LINX Resource"=w224:T7)  [unwired: 6 in]
                          n81 = flat-sequence {
                            tunnel: [w227] -> w219
                            tunnel: w220 -> [w227]
                            tunnel: w218 -> [w226]
                            frame #0 {
                              n82 = Wait (ms)(milliseconds to wait=w226) -> ()  [unwired: 1 out]
                            }
                          }
                        }
                        frame 7 {
                          n83 = call-poly <vilib>:"Digital Write.vi"("Error In"=w233, "Output Value"=TRUE, "DO Channel"=u8 26, "LINX Resource"=w235) -> ("Error Out"=w230:errorcluster, "LINX Resource"=w234:T7)  [unwired: 6 in]
                          n84 = flat-sequence {
                            tunnel: [w237] -> w229
                            tunnel: w230 -> [w237]
                            tunnel: w228 -> [w236]
                            frame #0 {
                              n85 = Wait (ms)(milliseconds to wait=w236) -> ()  [unwired: 1 out]
                            }
                          }
                        }
                        frame 9, Default {
                        }
                      }
                    }
                  }
                }
                frame True {
                }
              }
            }
          }
          frame "Read" {
            n86 = for {
              tunnel: [w343] -> w335 mode=indexing
              shift-right: [w341] -> w328
              shift-left: w334 -> [w342]
              tunnel: w333 -> [w337] mode=indexing
              tunnel: [w340] -> w321 mode=indexing
              shift-right: [w339] -> w327
              shift-left: w336 -> [w347]
              n87 = call "VL6180 GetDistance.vi"("Speed Read"="Speed Read", "VL6180 Resource in"=w337, "error in (no error)"=w347, "Attempts before Timeout"="Attempts before Timeout", "LINX Resource"=w342) -> ("error out"=w339:errorcluster, "Sensor Error Code"=→"Sensor Error Code":u8, "Distance (mm)"=w340:u8, "LINX Resource"=w341:T7, "Attempts"=→"Attempts":i32, "VL6180 Resource out"=w343:T21)  [unwired: 1 in]
            }
            n88 = Index Array(array=w321) -> (element #1=→"Gap 1":u8, element #2=→"Gap 2":u8, element #3=→"Gap 3":u8, element #4=→"Gap 4":u8, element #5=→"Rail Gap 1":u8, element #6=→"Rail Gap 2":u8)  [unwired: 6 in]
            n89 = local write "Status"("Reading Distances" ("Status")) -> ()
            n90 = local read "# of sensors"() -> (w325:i32)
            n91 = feedback-in #3(w325) -> ()
            n92 = feedback #3() -> (w324:i32)  [unwired: 1 in]
            n93 = Not Equal?(x=w324, y=w325) -> (x != y?=w326:bool)
            n94 = Or(x=w327, y=w326) -> (x .or. y?=w323:bool)
            n95 = Select(t=VL6180_states."Ping All", s=w323, f=VL6180_states."Read") -> (s? t:f=w332:T3)
          }
        }
        n96 = Wait (ms)(milliseconds to wait="Wait (ms)") -> ()  [unwired: 1 out]
      }
    }
    frame Error {
    }
  }
  n97 = node-c288(w18) -> ()  [unwired: 1 out]
  n98 = Compound Arithmetic op=OR(w12, w11, w10, w9, w8, w7, w6, w5) -> (w2:u16)
  n99 = disable-structure shown="Disabled" {
    disable-tunnel: u8[] [144, 0] ("Bytes to Write") -> [w353 _]
    disable-tunnel: [w352 _] -> w14
    disable-tunnel: [w350 _] -> w13
    frame Disabled {
      w352 = u8 72 ("Slave Address (7-bit)")
      n100 = xnode "I2C"("Slave Address (7-bit)"=w352, "Bytes to Write"=u8[] [1, 4, 131] ("Data")) -> ("error out"=w351:errorcluster)  [unwired: 1 in]
      n101 = xnode "I2C 2"("Slave Address (7-bit)"=w352, "Bytes to Write"=w353, "error in (no error)"=w351) -> ("error out"=w350:errorcluster)
    }
    frame Enabled {
    }
  }
  n102 = Split Number(x=w2) -> (hi(x)=w3:u8, lo(x)=w1:u8)
  n103 = Build Array(w3, w1) -> (w4:u8[])
  n104 = while {
    shift-right: [w441] -> _
    shift-left: w13 -> [w439]
    tunnel: w14 -> [w440]
    tunnel: w4 -> [w436]
    stop <- w450 stop-if-true
    n105 = xnode "Analog input (1 sample)"("error in (no error)"=w439) -> ("Voltage (A/AI1 (Pin 5))"=w446:dbl, "Current (A/AI0 (Pin 3))"=w445:dbl, "5V Regulator (A/AI2 (Pin 7))"=→"5V Regulator":dbl, "Stress (A/AI3 (Pin 9))"=w433:dbl, "error out"=w442:errorcluster)
    n106 = disable-structure shown="Disabled" {
      disable-tunnel: w436 -> [w456 _]
      disable-tunnel: [w455 _] -> w435
      disable-tunnel: u8 72 ("Slave Address (7-bit)") -> [w454 _]
      frame Disabled {
        n107 = xnode "I2C 3"("Slave Address (7-bit)"=w454, "Bytes to Write"=w456) -> ("error out"=w452:errorcluster)  [unwired: 1 in]
        n108 = flat-sequence {
          tunnel: w452 -> [w458]
          tunnel: [w458] -> w451
          frame #0 {
            n109 = Wait (ms)(milliseconds to wait=u32 1 ("Byte Count")) -> ()  [unwired: 1 out]
          }
        }
        n110 = xnode "Read ADC 2"("Slave Address (7-bit)"=w454, "Byte Count"=u32 2, "error in (no error)"=w451) -> ("Bytes Read"=w455:u8[])  [unwired: 1 out]
      }
      frame Enabled {
      }
    }
    n111 = disable-structure shown="Disabled" {
      disable-tunnel: w440 -> [w538 _]
      disable-tunnel: w439 -> [w537 _]
      disable-tunnel: [w536 _] -> _
      frame Disabled {
        n112 = xnode "Read ADC"("Slave Address (7-bit)"=w538, "Byte Count"=u32 2, "error in (no error)"=w537) -> ("Bytes Read"=w536:u8[])  [unwired: 1 out]
      }
      frame Enabled {
      }
    }
    n113 = call "power conversions.vi"("Current Raw"=w445, "Voltage Raw"=w446) -> ("Current"=→"Current":dbl, "Voltage"=→"Voltage":dbl)  [unwired: 8 in]
    n114 = Not(x="Sensor Power") -> (.not. x?=w443:bool)
    n115 = Subtract(x=5.0, y=w433) -> (x-y=→"Structure\nStress":dbl)
    n116 = local read "Wait (ms)"() -> (w438:u32)
    n117 = xnode "Digital output (1 sample)"("Sensor Power (B/DIO7 (Pin 25))"=w443, "error in (no error)"=w442) -> ("error out"=w441:errorcluster)
    n118 = call <vilib>:"Loop Frequency.vi"() -> ("Loop Rate (Hz)"=→"ToF Loop Rate":u32)
    n119 = Wait (ms)(milliseconds to wait=w438) -> ()  [unwired: 1 out]
    n120 = call "ADS1015 Raw2Formatted Converter.vi"("Bytes Read"=w435) -> ()  [unwired: 10 in, 1 out]
    n121 = local read "Stop"() -> (w450:bool)
  }
  n122 = flat-sequence {
    tunnel: w17 -> [w654]
    tunnel: [w654] -> w16
    frame #0 {
      n123 = local write "Stop"(FALSE ("Stop")) -> ()
    }
  }
  n124 = call <vilib>:"Close.vi"("Error In"=w16, "LINX Resource"=w20) -> ()  [unwired: 9 in, 1 out]
